vi "PseudoGellermann.vi"(10 "Start trues":i32=2 min=0 max=3, 11 "N":i32=10 min=10 step=2) -> (3 "Array":bool[](array[boolean]))   [LabVIEW 2013]
doc: "This VI creates an array of binary values, according to a pseudo Gellerman sequence"
panel:
  out "Iterations":i32
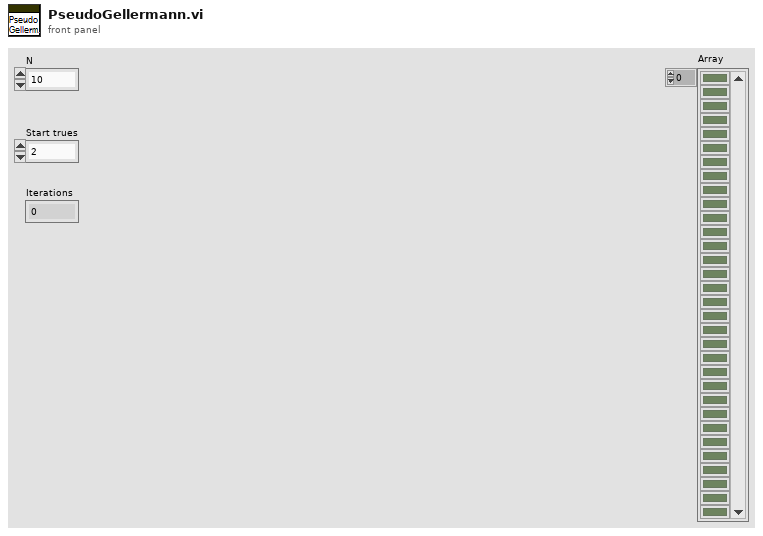
[diagram p1: front panel]
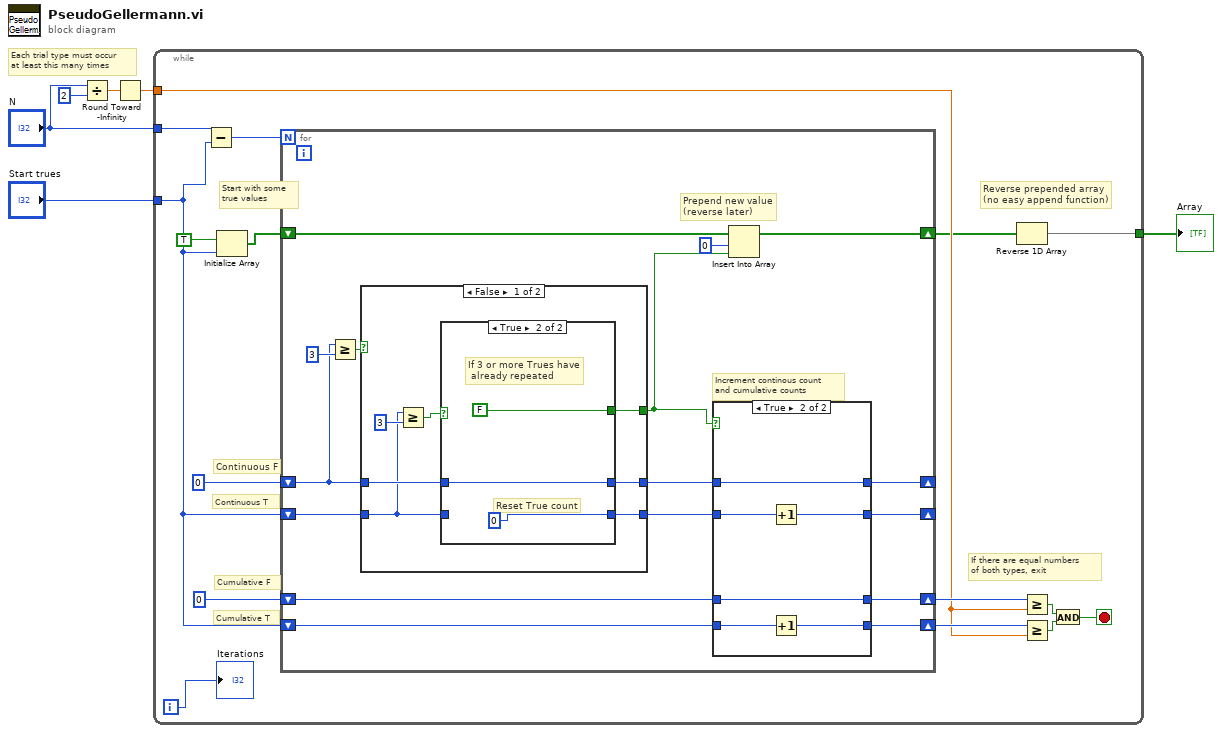
[diagram p0: block diagram]
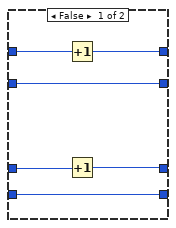
[diagram p2: hidden frame]
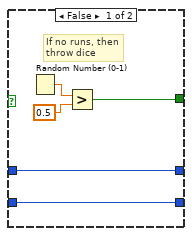
[diagram p3: hidden frame]
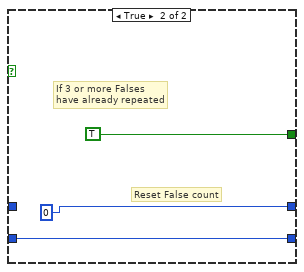
[diagram p4: hidden frame]
diagram:
  # "Each trial type must occur\nat least this many times"
  n1 = Divide(x="N", y=2) -> (x/y=w5:dbl)
  n2 = Round Toward -Infinity(1:w5) -> (0:w3:dbl)
  n3 = while {
    tunnel: "N" -> [w18]
    tunnel: w3 -> [w14]
    tunnel: [w9] -> w2
    tunnel: "Start trues" -> [w7]
    i -> [w10]
    stop <- w11 stop-if-true
    # "Reverse prepended array\n(no easy append function)"
    # "If there are equal numbers\nof both types, exit"
    # "Cumulative T"
    # "Cumulative F"
    # "Start with some\ntrue values"
    # "Continuous T"
    # "Continuous F"
    n4 = Subtract(x=w18, y=w7) -> (x-y=w17:i32)
    n5 = Initialize Array(TRUE, w7) -> (w20:bool[])
    n6 = for {
      N: w17 -> [_]
      shift-right: [w24] -> _
      shift-left: 0 ("dimension size") -> [w36]
      shift-right: [w26] -> _
      shift-left: w7 -> [w35]
      shift-right: [w32] -> w8
      shift-left: w20 -> [w34]
      shift-right: [w29] -> w16
      shift-left: 0 ("dimension size") -> [w31]
      shift-right: [w28] -> w15
      shift-left: w7 -> [w30]
      # "Increment continous count\nand cumulative counts"
      # "Prepend new value\n(reverse later)"
      n7 = Greater Or Equal?(x=w36, y=3) -> (x >= y?=w38:bool)
      n8 = case shown="False" w38 {
        tunnel: w36 -> [w55 _]
        tunnel: w35 -> [w51 w67]
        tunnel: [w54 w67] -> w27
        tunnel: [w53 0 ("dimension size")] -> w25
        tunnel: [w52 TRUE] -> w23
        frame False {
          n9 = Greater Or Equal?(x=w51, y=3) -> (x >= y?=w56:bool)
          n10 = case shown="True" w56 {
            tunnel: w55 -> [w59 w64]
            tunnel: [w58 0 ("dimension size")] -> w54
            tunnel: [w59 w64] -> w53
            tunnel: [w60 FALSE] -> w52
            tunnel: w51 -> [w58 _]
            frame False {
              # "If no runs, then\nthrow dice"
              n11 = Random Number (0-1)() -> (number: 0 to 1=w62:dbl)
              n12 = Greater?(x=w62, y=0.5) -> (0:w60:bool)
            }
            frame True {
              # "Reset True count"
              # "If 3 or more Trues have\n already repeated"
            }
          }
        }
        frame True {
          # "Reset False count"
          # "If 3 or more Falses \nhave already repeated"
        }
      }
      n13 = case shown="True" w23 {
        tunnel: w31 -> [w41 w48]
        tunnel: w30 -> [w39 w50]
        tunnel: [w40 w48] -> w29
        tunnel: [w39 w49] -> w28
        tunnel: w27 -> [w42 w47]
        tunnel: [w42 w46] -> w26
        tunnel: w25 -> [w44 w45]
        tunnel: [w43 w45] -> w24
        frame False {
          n14 = Increment(x=w44) -> (x+1=w43:i32)
          n15 = Increment(x=w41) -> (x+1=w40:i32)
        }
        frame True {
          n16 = Increment(x=w47) -> (x+1=w46:i32)
          n17 = Increment(x=w50) -> (x+1=w49:i32)
        }
      }
      n18 = Insert Into Array(array=w34, index=0, new element=w23) -> (w32:bool[])
    }
    n19 = Reverse 1D Array(array=w8) -> (reversed array=w9:bool[])
    n20 = Greater Or Equal?(x=w16, y=w14) -> (x >= y?=w12:bool)
    n21 = Greater Or Equal?(x=w15, y=w14) -> (x >= y?=w13:bool)
    n22 = And(x=w12, y=w13) -> (x .and. y?=w11:bool)
    "Iterations" <- w10
  }
  "Array" <- w2
